vi "File_PlayBack_PXDAC4800.vi"(4 "Length":u32, 5 "src_length_bytes":u32, 6 "Offset":u32, 7 "src_offset_bytes":u32, 8 "dst_length_bytes":u32, 9 "dst_offset_bytes":u32, 10 "NumBoard":u32=1) -> (0 "Error/output message":string, 1 "Serial num":u32, 2 "Status":i32, 3 "Handle":u32)   [LabVIEW 2016]
panel:
  in  "File":path
  # "LoadFileIntoRam options"
  # "BeginRamPlayback options"
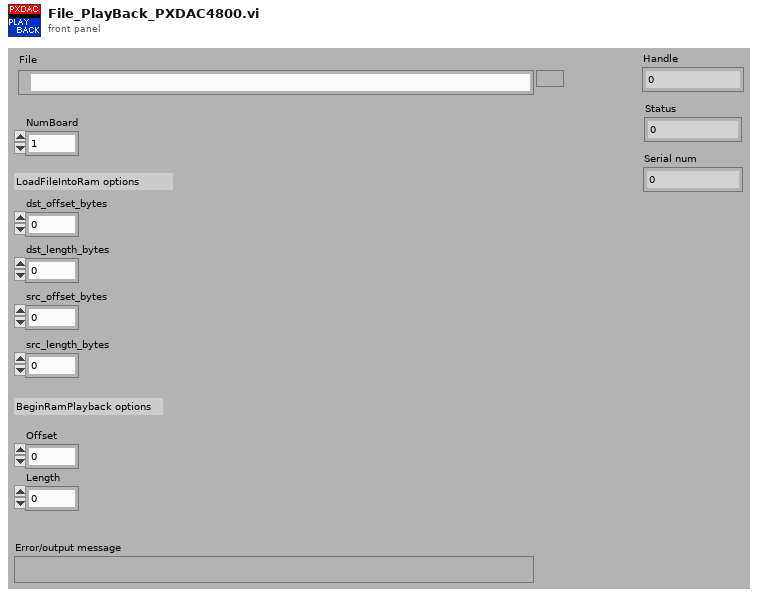
[diagram p1: front panel]
types:
  T1 = enum16{"Connect", "GetSerialNumber", "LoadFileIntoRam", "BeginRamPlayback", "Trigger", "EndRamPlaybackXD48", "Disconnect"}
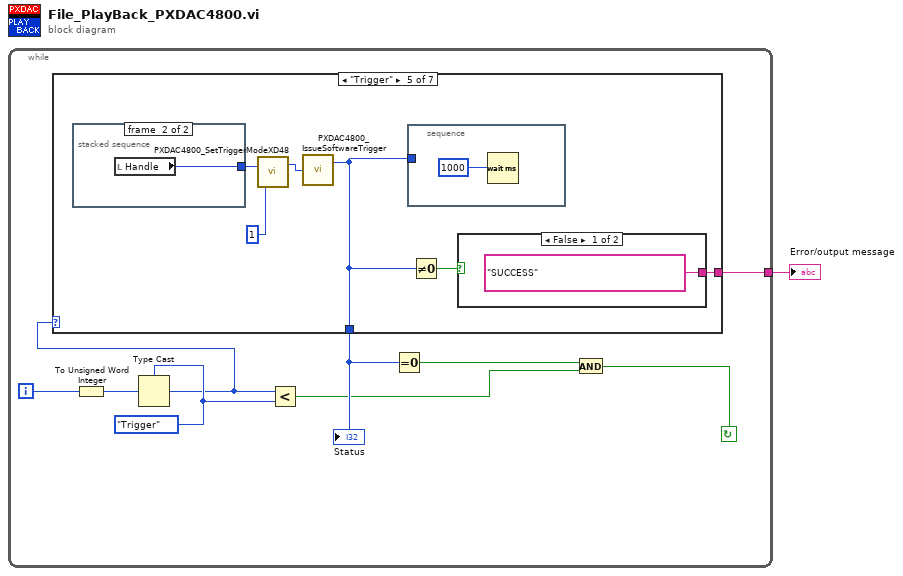
[diagram p0: block diagram]
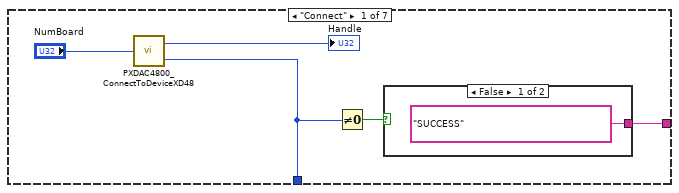
[diagram p2: hidden frame]
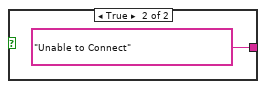
[diagram p3: hidden frame]
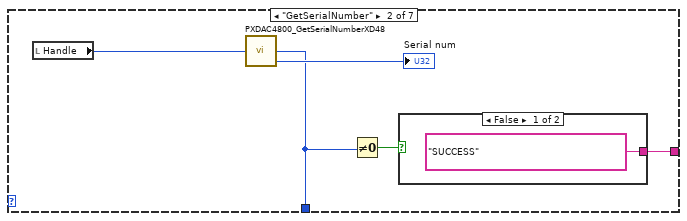
[diagram p4: hidden frame]
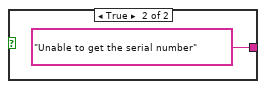
[diagram p5: hidden frame]
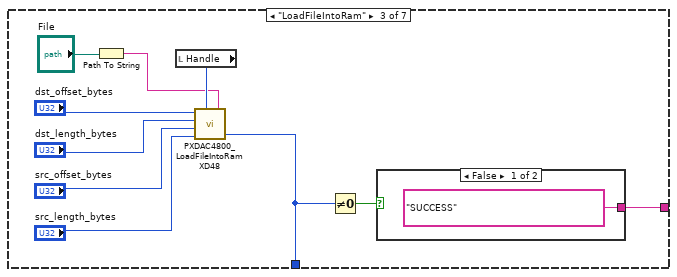
[diagram p6: hidden frame]
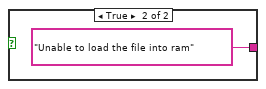
[diagram p7: hidden frame]
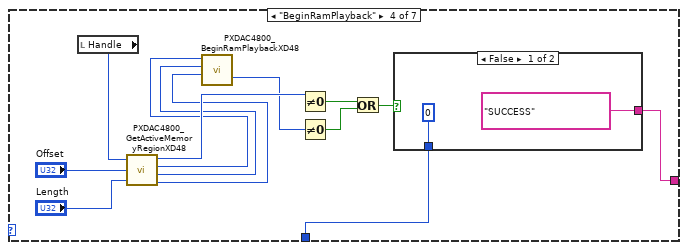
[diagram p8: hidden frame]
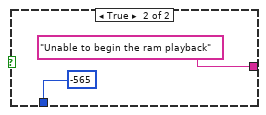
[diagram p9: hidden frame]
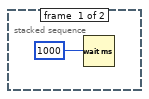
[diagram p10: hidden frame]
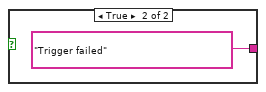
[diagram p11: hidden frame]
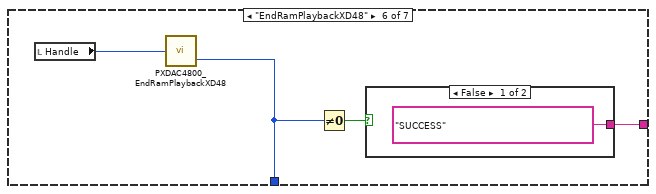
[diagram p12: hidden frame]
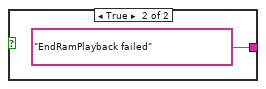
[diagram p13: hidden frame]
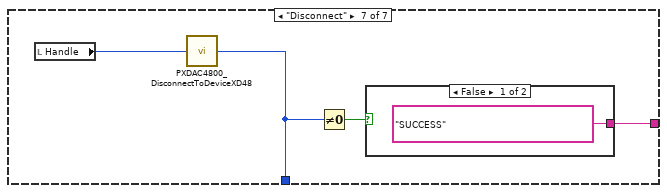
[diagram p14: hidden frame]
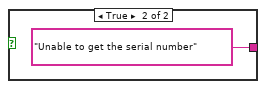
[diagram p15: hidden frame]
diagram:
  n1 = while {
    tunnel: [w3] -> w1
    i -> [w10]
    stop <- w4 continue-if-true
    w8 = T1."Trigger"
    n2 = To Unsigned Word Integer(number=w10) -> (unsigned 16bit integer=w9:u16)
    n3 = Type Cast(type=w8, x=w9) -> (*(type *) &x=w2:T1)
    n4 = case shown="\"Trigger\"" w2 {
      tunnel: [w11 w18 w28 w47 w57 w65 w71] -> w7
      tunnel: [w14 w21 w34 w49 w58 w67 w74] -> w3
      frame "Connect" {
        n5 = call "PXDAC4800_ConnectToDeviceXD48.vi"("brdNum"="NumBoard") -> ("Handle Out"=→"Handle":i32, "Status"=w11:i32)
        n6 = Not Equal To 0?(x=w11) -> (x != 0?=w15:bool)
        n7 = case shown="False" w15 {
          tunnel: ["SUCCESS" "Unable to Connect"] -> w14
          frame False {
          }
          frame True {
          }
        }
      }
      frame "GetSerialNumber" {
        (unwired) "Unable to get serial"
        n8 = local read "Handle"() -> (w20:u32)
        n9 = call "PXDAC4800_GetSerialNumberXD48.vi"("Handle"=w20) -> ("Status"=w18:i32, "Serial num"=→"Serial num":i32)  [unwired: 1 out]
        n10 = Not Equal To 0?(x=w18) -> (x != 0?=w22:bool)
        n11 = case shown="False" w22 {
          tunnel: ["SUCCESS" "Unable to get the serial number"] -> w21
          frame False {
          }
          frame True {
          }
        }
      }
      frame "LoadFileIntoRam" {
        n12 = Path To String(path="File") -> (string=w25:string)
        n13 = local read "Handle"() -> (w27:u32)
        n14 = call "PXDAC4800_LoadFileIntoRamXD48.vi"("dst_offset_bytes"="dst_offset_bytes", "Handle"=w27, "dst_length_bytes"="dst_length_bytes", "src_offset_bytes"="src_offset_bytes", "src_length_bytes"="src_length_bytes", "File_Path"=w25) -> ("Status"=w28:i32)  [unwired: 1 in, 1 out]
        n15 = Not Equal To 0?(x=w28) -> (x != 0?=w33:bool)
        n16 = case shown="False" w33 {
          tunnel: ["SUCCESS" "Unable to load the file into ram"] -> w34
          frame False {
          }
          frame True {
          }
        }
      }
      frame "BeginRamPlayback" {
        n17 = local read "Handle"() -> (w37:u32)
        n18 = call "PXDAC4800_GetActiveMemoryRegionXD48.vi"("Handle"=w37, "Offset"="Offset", "Length Byte"="Length") -> ("Status"=w44:i32, "Handle out"=w43:u32, "Offset_bytes out"=w42:u32, "Playback_bytes out"=w41:u32)
        n19 = call "PXDAC4800_BeginRamPlaybackXD48.vi"("ram length bytes"=w41, "ram offset bytes"=w42, "Handle"=w43) -> ("Status"=w38:i32)  [unwired: 1 in, 1 out]
        n20 = Not Equal To 0?(x=w44) -> (x != 0?=w48:bool)
        n21 = Not Equal To 0?(x=w38) -> (x != 0?=w46:bool)
        n22 = Or(x=w48, y=w46) -> (x .or. y?=w45:bool)
        n23 = case shown="False" w45 {
          tunnel: ["SUCCESS" "Unable to begin the ram playback"] -> w49
          tunnel: [0 -565] -> w47
          frame False {
          }
          frame True {
          }
        }
      }
      frame "Trigger" {
        n24 = stacked-sequence {
          tunnel: [_ w62] -> w56
          frame #0 {
            n25 = Wait (ms)(milliseconds to wait=1000) -> ()  [unwired: 1 out]
          }
          frame #1 {
            n26 = local read "Handle"() -> (w62:u32)
          }
        }
        n27 = call "PXDAC4800_SetTriggerModeXD48.vi"("Value"=1, "Handle"=w56) -> ("Handle out"=w54:u32)  [unwired: 1 out]
        n28 = call "PXDAC4800_IssueSoftwareTrigger.vi"("Handle"=w54) -> ("Status"=w57:i32)  [unwired: 1 out]
        n29 = stacked-sequence {
          tunnel: w57 -> [_]
          frame #0 {
            n30 = Wait (ms)(milliseconds to wait=1000) -> ()  [unwired: 1 out]
          }
        }
        n31 = Not Equal To 0?(x=w57) -> (x != 0?=w59:bool)
        n32 = case shown="False" w59 {
          tunnel: ["SUCCESS" "Trigger failed"] -> w58
          frame False {
          }
          frame True {
          }
        }
      }
      frame "EndRamPlaybackXD48" {
        n33 = local read "Handle"() -> (w66:u32)
        n34 = call "PXDAC4800_EndRamPlaybackXD48.vi"("Handle"=w66) -> ("Status"=w65:i32)  [unwired: 1 out]
        n35 = Not Equal To 0?(x=w65) -> (x != 0?=w68:bool)
        n36 = case shown="False" w68 {
          tunnel: ["SUCCESS" "EndRamPlayback failed"] -> w67
          frame False {
          }
          frame True {
          }
        }
      }
      frame "Disconnect" {
        n37 = local read "Handle"() -> (w72:u32)
        n38 = call "PXDAC4800_DisconnectToDeviceXD48.vi"("Handle"=w72) -> ("Status"=w71:i32)
        n39 = Not Equal To 0?(x=w71) -> (x != 0?=w73:bool)
        n40 = case shown="False" w73 {
          tunnel: ["SUCCESS" "Unable to get the serial number"] -> w74
          frame False {
          }
          frame True {
          }
        }
      }
    }
    "Status" <- w7
    n41 = Less?(x=w2, y=w8) -> (x < y?=w5:bool)
    n42 = Equal To 0?(x=w7) -> (x = 0?=w6:bool)
    n43 = And(x=w6, y=w5) -> (x .and. y?=w4:bool)
  }
  "Error/output message" <- w1
